vi "Write Document Source.vi"(8 "error in (no error)":errorcluster, 10 "Value":string, 11 "WebView2 Control in":refnum<class "WebView2 QControl.lvclass">) -> (0 "error out":errorcluster, 3 "WebView2 Control out":refnum<class "WebView2 QControl.lvclass">)   [LabVIEW 2020, in "WebView2 QControl.lvlib" / "WebView2 QControl.lvclass"]
uses:
  WebView2 QControl.lvclass
  WebView2 QControl.lvclass/WebView2 QControl.ctl
  Webview2 Lib/WebView2 Control Object/WebView2 Control.lvclass
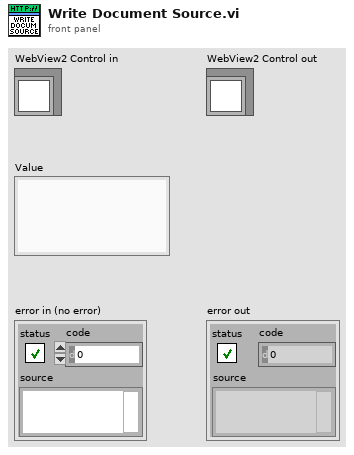
[diagram p1: front panel]
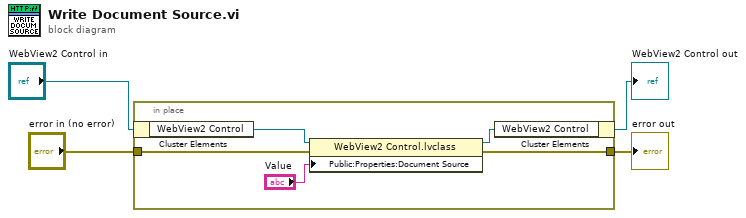
[diagram p0: block diagram]
diagram:
  n1 = in-place {
    in-place-border: [w9] -> w1
    in-place-border: "error in (no error)" -> [w6]
    n2 = in-place-cluster #1("WebView2 Control in") -> ("WebView2 Control"=w8:refnum<class "WebView2 Control.lvclass">)
    n3 = property class="WebView2 Control.lvclass"(reference=w8, error in=w6, "Public:Properties:Document Source"="Value") -> (reference out=w7:refnum<class "WebView2 Control.lvclass">, error out=w9:errorcluster)
    n4 = in-place-cluster #1("WebView2 Control"=w7) -> (→"WebView2 Control out":refnum<class "WebView2 QControl.lvclass">)
  }
  "error out" <- w1
